vi "Sensor Interface View.vi"(8 "error in (no error)":errorcluster, 11 "View Model":T1) -> (0 "error out":errorcluster)   [LabVIEW 2017]
doc: "Interface for simulation the depositing of checks or cash and dispensing of cash.\n[Covers: UI4]"
uses:
  View Model/Controls/View Model.ctl
  Error Handler/Controls/Error Model.ctl
  Error Handler/Controls/Error Data.ctl
  Error Handler/Controls/Error Type.ctl
  View Model/Controls/Shared Model.ctl
  Configuration/Controls/Config Model.ctl
  Configuration/Controls/Config CMD.ctl
  Configuration/Controls/Config Data.ctl
  ATM Controller/Controls/Controller Model.ctl
  ATM Controller/Controls/Controller Overhead.ctl
  ATM Controller/Controls/Controller States.ctl
  User Console View/Controls/User Console - Keypad.ctl
  User Console View/Controls/User Console - Transactions.ctl
  ATM Controller/Controls/Controller CMD.ctl
panel:
  in  "Funds Dispensed":bool
  in  "Deposit Received":bool
  # "[Covers: UI4A]"
  # "[Covers: UI4B]"
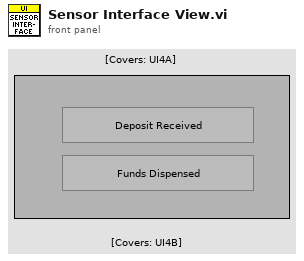
[diagram p1: front panel]
types:
  T1 = typedef "View Model.ctl" = cluster{"Error Model":T2, "Shared Model":T3, "Config Model":T4, "Controller Model":T5}
  T2 = typedef "Error Model.ctl" = cluster{"Error Event":refnum<user-event>}
  T3 = typedef "Shared Model.ctl" = cluster{"Stop Event":refnum<user-event>, "Stop DVR":refnum<data-value>}
  T4 = typedef "Config Model.ctl" = cluster{"Config CMD":refnum<user-event>, "Config Data DVR":refnum<data-value>}
  T5 = typedef "Controller Model.ctl" = cluster{"Controller Overhead DVR":refnum<data-value>, "Deposit Received Change":refnum<user-event>, "Fund Transaction Change":refnum<user-event>, "Card Read Change":refnum<user-event>, "Keypad Change":refnum<user-event>, "Transaction Change":refnum<user-event>, "Controller CMD Change":refnum<user-event>}
  T6 = enum8{"Enabled", "Disabled", "Disabled and Grayed Out"}
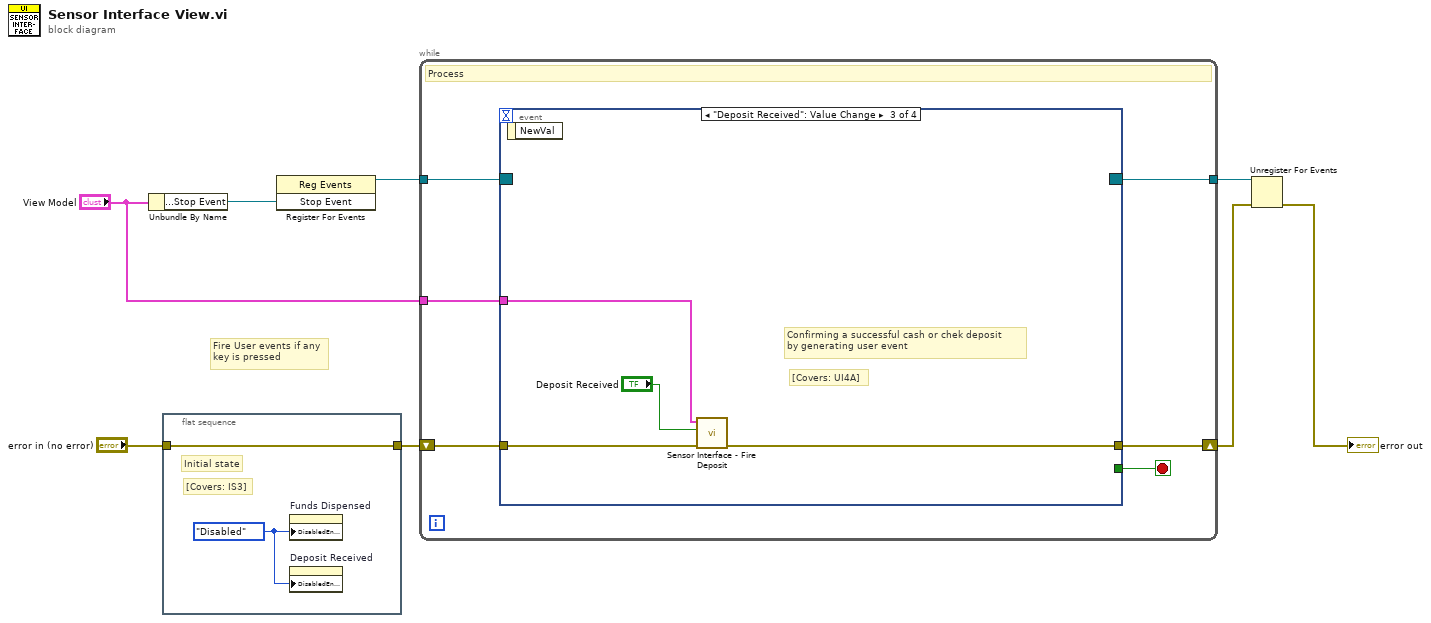
[diagram p0: block diagram]
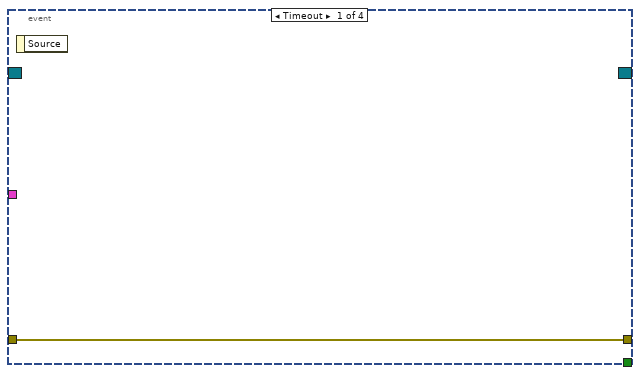
[diagram p2: hidden frame]
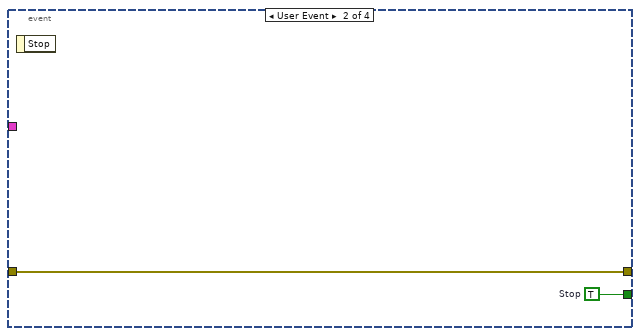
[diagram p3: hidden frame]
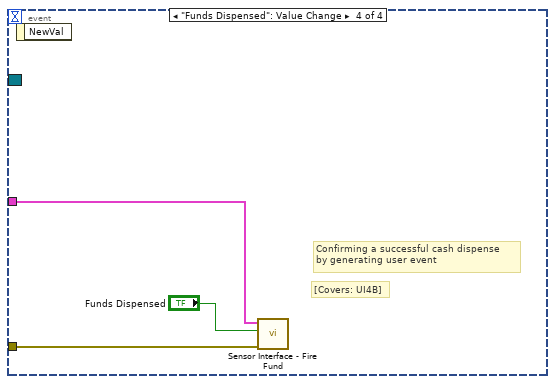
[diagram p4: hidden frame]
diagram:
  # "Fire User events if any\nkey is pressed"
  n1 = Unbundle By Name("View Model") -> ("Shared Model.Stop Event"=w8:refnum<user-event>)
  n2 = flat-sequence {
    tunnel: "error in (no error)" -> [w9]
    tunnel: [w9] -> w1
    frame #0 {
      w10 = T6."Disabled" ("Disabled")
      # "[Covers: IS3]"
      # "Initial state"
      n3 = property on="Funds Dispensed" class="Bool"("DisabledEnum"=w10) -> ()  [unwired: 2 in, 2 out]
      n4 = property on="Deposit Received" class="Bool"("DisabledEnum"=w10) -> ()  [unwired: 2 in, 2 out]
    }
  }
  n5 = register-events(w8) -> (reference out=w7:refnum<event-registration>)  [unwired: 2 in, 1 out]
  n6 = while {
    tunnel: w7 -> [w16]
    shift-right: [w13] -> w5
    shift-left: w1 -> [w14]
    tunnel: [w12] -> w6
    tunnel: "View Model" -> [w11]
    stop <- w15 stop-if-true
    # "Process"
    n7 = event shown="[2] \"Deposit Received\": Value Change" {
      selector: w16 -> [_ _ _ _]
      dyn-events: [_ _ _ _] -> w12
      timeout: _ -> [_ _ _ _]
      tunnel: [_ w19 _ _] -> w15
      tunnel: w14 -> [w17 w18 w23 w26]
      tunnel: [w17 w18 w20 _] -> w13
      tunnel: w11 -> [_ _ w22 w25]
      event Timeout {
        n8 = event-data() -> ()  [unwired: 1 in, 1 out]
      }
      event User Event {
        w19 = TRUE  # Stop
        n9 = event-data() -> ()  [unwired: 1 in, 1 out]
      }
      event "Deposit Received": Value Change {
        # "[Covers: UI4A]"
        # "Confirming a successful cash or chek deposit\nby generating user event"
        n10 = event-data() -> ()  [unwired: 1 in, 1 out]
        n11 = call "Sensor Interface - Fire Deposit.vi"("error in (no error)"=w23, "Deposit Received"="Deposit Received", "View Model"=w22) -> ("error out"=w20:errorcluster)  [unwired: 7 in, 1 out]
      }
      event "Funds Dispensed": Value Change {
        # "[Covers: UI4B]"
        # "Confirming a successful cash dispense\nby generating user event"
        n12 = event-data() -> ()  [unwired: 1 in, 1 out]
        n13 = call "Sensor Interface - Fire Fund.vi"("error in (no error)"=w26, "Fund Transaction"="Funds Dispensed", "View Model"=w25) -> ()  [unwired: 7 in, 2 out]
      }
    }
  }
  n14 = Unregister For Events(event registration refnum=w6, error in=w5) -> (error out=→"error out":errorcluster)
